vi "Write Model constants.vi"(10 "Model constants":T1, 11 "CurrentToField in":refnum<class "CurrentToField.lvclass">) -> (3 "CurrentToField out":refnum<class "CurrentToField.lvclass">)   [LabVIEW 2019, in "CurrentToField.lvclass"]
uses:
  CurrentToField.lvclass
  CurrentToField.lvclass/CurrentToField.ctl
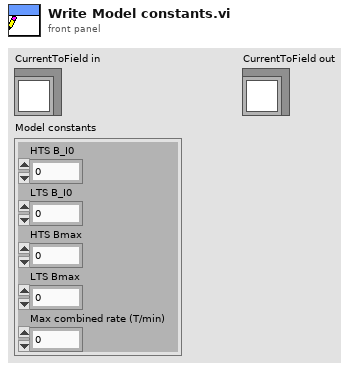
[diagram p1: front panel]
types:
  T1 = cluster{"HTS B_I0":dbl, "LTS B_I0":dbl, "HTS Bmax":dbl, "LTS Bmax":dbl, "Max combined rate (T/min)":dbl}
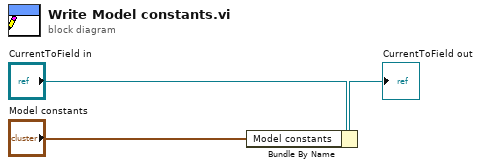
[diagram p0: block diagram]
diagram:
  n1 = Bundle By Name(cluster="CurrentToField in", "Model constants"="Model constants") -> (→"CurrentToField out":refnum<class "CurrentToField.lvclass">)
